vi "Tree_GetAll.vi"(8 "Error In":errorcluster, 11 "Tree Refnum IN":refnum<vi>) -> (0 "Error Out":errorcluster, 1 "Text":string[](array[string]), 2 "Tags":string[](array[string]), 3 "Tree Refnum OUT":refnum<vi>)   [LabVIEW 2012]
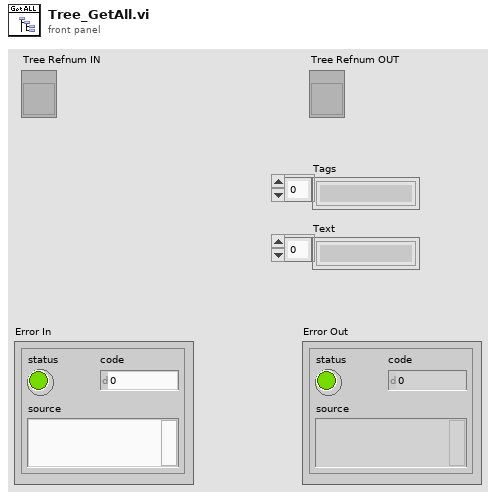
[diagram p1: front panel]
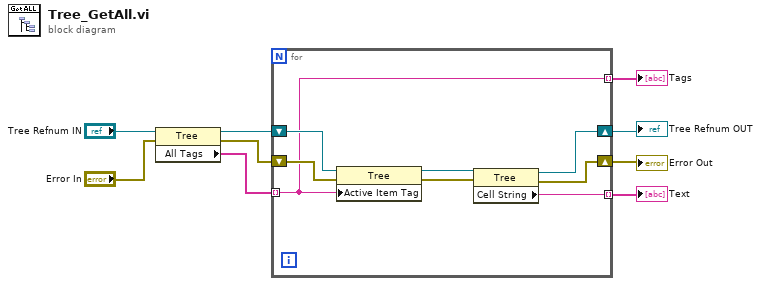
[diagram p0: block diagram]
diagram:
  n1 = property class="Tree"(reference="Tree Refnum IN", error in="Error In") -> (reference out=w8:refnum<vi>, error out=w7:errorcluster, "All Tags"=w9:string[])
  n2 = for {
    tunnel: w9 -> [w10] mode=indexing
    shift-right: [w11] -> w1
    shift-left: w8 -> [w14]
    shift-right: [w12] -> w2
    shift-left: w7 -> [w15]
    tunnel: [w13] -> w6 mode=indexing
    tunnel: [w10] -> w5 mode=indexing
    n3 = property class="Tree"(reference=w14, error in=w15, "Active Item Tag"=w10) -> (reference out=w17:refnum<vi>, error out=w16:errorcluster)
    n4 = property class="Tree"(reference=w17, error in=w16) -> (reference out=w11:refnum<vi>, error out=w12:errorcluster, "Cell String"=w13:string)
  }
  "Text" <- w6
  "Tags" <- w5
  "Tree Refnum OUT" <- w1
  "Error Out" <- w2
